vi "draw_gameplay.vi"(10 "status":T1={"player1"={"x"=0, "y"=180, "dive_direction"=-1, "state"=3, "frame_num"=0}, "player2"={"x"=300, "y"=180, "state"=3, "frame_num"=0, "dive_direction"=-1}, "ball"={"x"=150, "y"=100, "rotation"=1}, "ball_hyper"={"x"=100, "y"=100, "visible"=TRUE}, "ball_trail"={"x"=200, "y"=100, "visible"=TRUE}, "punch"={"x"=150, "y"=100, "visible"=TRUE}}, 11 "input":picture) -> (3 "gameplay":picture)   [LabVIEW 2025]
uses:
  <vilib>/Utility/miscctls.llb/LVBoundsTypeDef.ctl
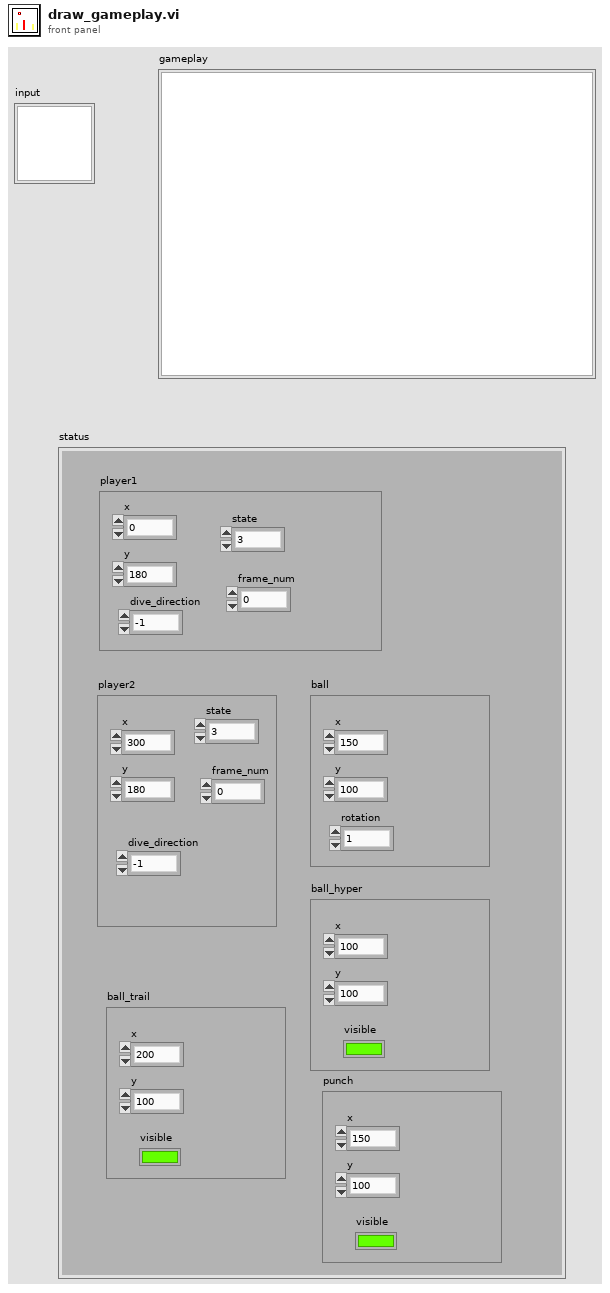
[diagram p1: front panel]
types:
  T1 = cluster{"player1":cluster{"x":i32, "y":i32, "dive_direction":i32, "state":i32, "frame_num":i32}, "player2":cluster{"x":i32, "y":i32, "state":i32, "frame_num":i32, "dive_direction":i32}, "ball":cluster{"x":i32, "y":i32, "rotation":i32}, "ball_hyper":cluster{"x":i32, "y":i32, "visible":bool}, "ball_trail":cluster{"x":i32, "y":i32, "visible":bool}, "punch":cluster{"x":i32, "y":i32, "visible":bool}}
  T2 = typedef "LVBoundsTypeDef.ctl" = cluster{"Width":u32, "Height":u32}
  T3 = cluster{"x":i32, "y":i32, "dive_direction":i32, "state":i32, "frame_num":i32}
  T4 = cluster{"x":i32, "y":i32, "state":i32, "frame_num":i32, "dive_direction":i32}
  T5 = typedef "imagedata.ctl" = cluster{"image type":i32, "image depth":i32, "image":u8[], "mask":u8[], "colors":u32[], "Rectangle":cluster{"left":i16, "top":i16, "right":i16, "bottom":i16}}
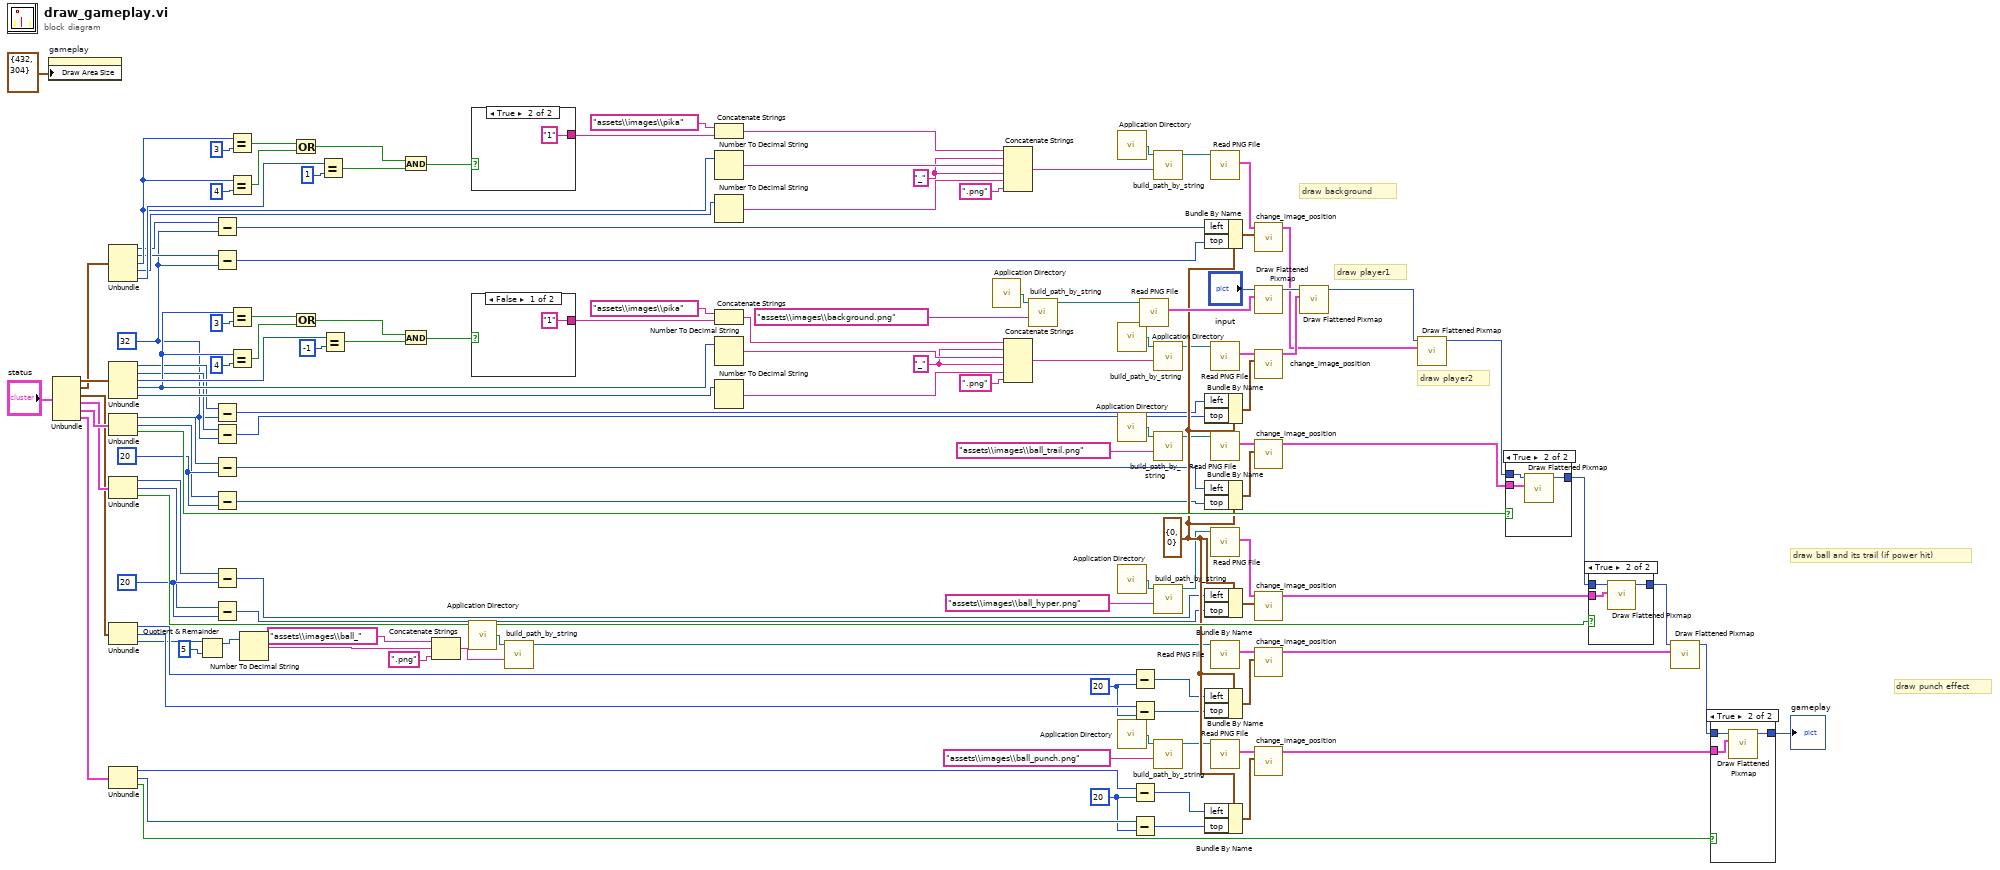
[diagram p0: block diagram]
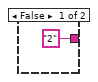
[diagram p5: hidden frame]
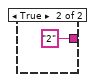
[diagram p6: hidden frame]
diagram:
  w29 = 20
  w35 = 20
  w40 = 20
  w43 = 20
  w49 = 32 ("y")
  w82 = "_"
  w113 = "_"
  w58 = cluster{"left":i32, "top":i32} {"left"=0, "top"=0} ("position")
  # "draw punch effect"
  # "draw background"
  # "draw ball and its trail (if power hit)"
  # "draw player2"
  # "draw player1"
  n1 = property on="gameplay" class="Pict"("Draw Area Size"=T2 {"Width"=432, "Height"=304}) -> ()  [unwired: 2 in, 2 out]
  n2 = Unbundle("status") -> ("player1"=w118:T3, "player2"=w117:T4, "ball"=w68:cluster{"x":i32, "y":i32, "rotation":i32}, "ball_hyper"=w71:cluster{"x":i32, "y":i32, "visible":bool}, "ball_trail"=w80:cluster{"x":i32, "y":i32, "visible":bool}, "punch"=w57:cluster{"x":i32, "y":i32, "visible":bool})
  n3 = Unbundle(w117) -> ("x"=w54:i32, "y"=w50:i32, "state"=w85:i32, "frame_num"=w84:i32, "dive_direction"=w88:i32)
  n4 = Unbundle(w118) -> ("x"=w56:i32, "y"=w53:i32, "dive_direction"=w107:i32, "state"=w102:i32, "frame_num"=w116:i32)
  n5 = Unbundle(w80) -> ("x"=w34:i32, "y"=w33:i32, "visible"=w79:bool)
  n6 = Unbundle(w71) -> ("x"=w30:i32, "y"=w28:i32, "visible"=w75:bool)
  n7 = Unbundle(w68) -> ("x"=w42:i32, "y"=w41:i32, "rotation"=w3:i32)
  n8 = Unbundle(w57) -> ("x"=w47:i32, "y"=w46:i32, "visible"=w61:bool)
  n9 = Quotient & Remainder(x=w3, y=5) -> (x-y*floor(x/y)=w2:i32)  [unwired: 1 out]
  n10 = Subtract(x=w54, y=w49) -> (x-y=w51:i32)
  n11 = Subtract(x=w50, y=w49) -> (x-y=w48:i32)
  n12 = Subtract(x=w56, y=w49) -> (x-y=w55:i32)
  n13 = Subtract(x=w53, y=w49) -> (x-y=w52:i32)
  n14 = Subtract(x=w34, y=w35) -> (x-y=w31:i32)
  n15 = Subtract(x=w33, y=w35) -> (x-y=w32:i32)
  n16 = Subtract(x=w30, y=w29) -> (x-y=w27:i32)
  n17 = Subtract(x=w28, y=w29) -> (x-y=w26:i32)
  n18 = Equal?(x=w85, y=3) -> (x = y?=w95:bool)
  n19 = Equal?(x=w85, y=4) -> (x = y?=w96:bool)
  n20 = Equal?(x=w102, y=3) -> (x = y?=w104:bool)
  n21 = Equal?(x=w102, y=4) -> (x = y?=w103:bool)
  n22 = Number To Decimal String(number=w2) -> (decimal integer string=w65:string)  [unwired: 1 in]
  n23 = Or(x=w95, y=w96) -> (x .or. y?=w94:bool)
  n24 = Or(x=w104, y=w103) -> (x .or. y?=w105:bool)
  n25 = Equal?(x=w88, y=1) -> (x = y?=w91:bool)
  n26 = Equal?(x=w107, y=-1) -> (x = y?=w109:bool)
  n27 = And(x=w94, y=w91) -> (x .and. y?=w92:bool)
  n28 = And(x=w105, y=w109) -> (x .and. y?=w108:bool)
  n29 = Concatenate Strings("assets\\images\\ball_", w65, ".png" ("string")) -> (w8:string)
  n30 = call <vilib>:"Application Directory.vi"() -> ("Application Directory"=w9:path)
  n31 = case shown="True" w92 {
    tunnel: ["2" "1"] -> w90
    frame False {
    }
    frame True {
    }
  }
  n32 = case shown="False" w108 {
    tunnel: ["1" "2"] -> w110
    frame False {
    }
    frame True {
    }
  }
  n33 = call "build_path_by_string.vi"("String"=w8, "base path"=w9) -> ("appended path"=w7:path)  [unwired: 9 in]
  n34 = Concatenate Strings("assets\\images\\pika", w90) -> (w87:string)
  n35 = Number To Decimal String(number=w85) -> (decimal integer string=w83:string)  [unwired: 1 in]
  n36 = Number To Decimal String(number=w84) -> (decimal integer string=w81:string)  [unwired: 1 in]
  n37 = Concatenate Strings("assets\\images\\pika", w110) -> (w99:string)
  n38 = Number To Decimal String(number=w102) -> (decimal integer string=w114:string)  [unwired: 1 in]
  n39 = Number To Decimal String(number=w116) -> (decimal integer string=w115:string)  [unwired: 1 in]
  n40 = call <vilib>:"Application Directory.vi"() -> ("Application Directory"=w24:path)
  n41 = Concatenate Strings(w87, w82, w83, w82, w81, ".png" ("string")) -> (w17:string)
  n42 = Concatenate Strings(w99, w113, w114, w113, w115, ".png" ("string")) -> (w19:string)
  n43 = call "build_path_by_string.vi"("String"="assets\\images\\background.png", "base path"=w24) -> ("appended path"=w22:path)  [unwired: 9 in]
  n44 = call <vilib>:"Application Directory.vi"() -> ("Application Directory"=w18:path)
  n45 = call <vilib>:"Application Directory.vi"() -> ("Application Directory"=w21:path)
  n46 = call <vilib>:"Application Directory.vi"() -> ("Application Directory"=w15:path)
  n47 = call <vilib>:"Application Directory.vi"() -> ("Application Directory"=w12:path)
  n48 = call <vilib>:"Application Directory.vi"() -> ("Application Directory"=w6:path)
  n49 = Subtract(x=w42, y=w40) -> (x-y=w39:i32)
  n50 = Subtract(x=w41, y=w40) -> (x-y=w38:i32)
  n51 = Subtract(x=w47, y=w43) -> (x-y=w45:i32)
  n52 = Subtract(x=w46, y=w43) -> (x-y=w44:i32)
  n53 = call <vilib>:"Read PNG File.vi"("path to PNG file"=w22) -> ("image data"=w130:T5)  [unwired: 8 in, 2 out]
  n54 = call "build_path_by_string.vi"("String"=w17, "base path"=w18) -> ("appended path"=w16:path)  [unwired: 9 in]
  n55 = call "build_path_by_string.vi"("String"=w19, "base path"=w21) -> ("appended path"=w20:path)  [unwired: 9 in]
  n56 = call "build_path_by_string.vi"("String"="assets\\images\\ball_trail.png", "base path"=w15) -> ("appended path"=w14:path)  [unwired: 9 in]
  n57 = call "build_path_by_string.vi"("String"="assets\\images\\ball_hyper.png", "base path"=w12) -> ("appended path"=w11:path)  [unwired: 9 in]
  n58 = call "build_path_by_string.vi"("String"="assets\\images\\ball_punch.png", "base path"=w6) -> ("appended path"=w5:path)  [unwired: 9 in]
  n59 = Bundle By Name(cluster=w58, "left"=w51, "top"=w48) -> (w120:cluster{"left":i32, "top":i32})
  n60 = Bundle By Name(cluster=w58, "left"=w55, "top"=w52) -> (w121:cluster{"left":i32, "top":i32})
  n61 = Bundle By Name(cluster=w58, "left"=w31, "top"=w32) -> (w119:cluster{"left":i32, "top":i32})
  n62 = Bundle By Name(cluster=w58, "left"=w27, "top"=w26) -> (w74:cluster{"left":i32, "top":i32})
  n63 = Bundle By Name(cluster=w58, "left"=w39, "top"=w38) -> (w69:cluster{"left":i32, "top":i32})
  n64 = Bundle By Name(cluster=w58, "left"=w45, "top"=w44) -> (w62:cluster{"left":i32, "top":i32})
  n65 = call <vilib>:"Read PNG File.vi"("path to PNG file"=w16) -> ("image data"=w124:T5)  [unwired: 8 in, 2 out]
  n66 = call <vilib>:"Read PNG File.vi"("path to PNG file"=w20) -> ("image data"=w128:T5)  [unwired: 8 in, 2 out]
  n67 = call <vilib>:"Read PNG File.vi"("path to PNG file"=w14) -> ("image data"=w122:T5)  [unwired: 8 in, 2 out]
  n68 = call <vilib>:"Read PNG File.vi"("path to PNG file"=w11) -> ("image data"=w73:T5)  [unwired: 8 in, 2 out]
  n69 = call <vilib>:"Read PNG File.vi"("path to PNG file"=w7) -> ("image data"=w70:T5)  [unwired: 8 in, 2 out]
  n70 = call <vilib>:"Read PNG File.vi"("path to PNG file"=w5) -> ("image data"=w63:T5)  [unwired: 8 in, 2 out]
  n71 = call "change_image_position.vi"("position"=w120, "image data in"=w124) -> ("image data out"=w123:T5)  [unwired: 9 in]
  n72 = call <vilib>:"Draw Flattened Pixmap.vi"("image data"=w130, "picture"="input") -> ("new picture"=w126:picture)  [unwired: 7 in]
  n73 = call "change_image_position.vi"("position"=w121, "image data in"=w128) -> ("image data out"=w127:T5)  [unwired: 9 in]
  n74 = call "change_image_position.vi"("position"=w119, "image data in"=w122) -> ("image data out"=w78:T5)  [unwired: 9 in]
  n75 = call "change_image_position.vi"("position"=w74, "image data in"=w73) -> ("image data out"=w76:T5)  [unwired: 9 in]
  n76 = call "change_image_position.vi"("position"=w69, "image data in"=w70) -> ("image data out"=w36:T5)  [unwired: 9 in]
  n77 = call "change_image_position.vi"("position"=w62, "image data in"=w63) -> ("image data out"=w37:T5)  [unwired: 9 in]
  n78 = call <vilib>:"Draw Flattened Pixmap.vi"("image data"=w127, "picture"=w126) -> ("new picture"=w125:picture)  [unwired: 7 in]
  n79 = call <vilib>:"Draw Flattened Pixmap.vi"("image data"=w123, "picture"=w125) -> ("new picture"=w77:picture)  [unwired: 7 in]
  n80 = case shown="True" w79 {
    tunnel: w78 -> [_ w139]
    tunnel: w77 -> [w136 w138]
    tunnel: [w136 w137] -> w72
    frame False {
    }
    frame True {
      n81 = call <vilib>:"Draw Flattened Pixmap.vi"("image data"=w139, "picture"=w138) -> ("new picture"=w137:picture)  [unwired: 7 in]
    }
  }
  n82 = case shown="True" w75 {
    tunnel: w76 -> [_ w143]
    tunnel: w72 -> [w140 w142]
    tunnel: [w140 w141] -> w67
    frame False {
    }
    frame True {
      n83 = call <vilib>:"Draw Flattened Pixmap.vi"("image data"=w143, "picture"=w142) -> ("new picture"=w141:picture)  [unwired: 7 in]
    }
  }
  n84 = call <vilib>:"Draw Flattened Pixmap.vi"("image data"=w36, "picture"=w67) -> ("new picture"=w60:picture)  [unwired: 7 in]
  n85 = case shown="True" w61 {
    tunnel: w37 -> [_ w147]
    tunnel: w60 -> [w144 w146]
    tunnel: [w144 w145] -> w59
    frame False {
    }
    frame True {
      n86 = call <vilib>:"Draw Flattened Pixmap.vi"("image data"=w147, "picture"=w146) -> ("new picture"=w145:picture)  [unwired: 7 in]
    }
  }
  "gameplay" <- w59
